vi "Example_GameWithVisual.vi"() -> ()   [LabVIEW 2015]
uses:
  TronviewGame/Game/GameResult.ctl
  TronviewGame/Board/BoardSize.ctl
  TronviewPresentation/BoardDisplay/BoardDisplay.lvclass
  TronviewGame/Game/Game.lvclass/Game.ctl
  TronviewGame/Game/GetGameRecorder.vi
  TronviewGame/GameRecorder/GameRecorder.lvclass
  TronviewGame/Board/Board.lvclass
  TronviewGame/Game/Game.lvclass
  TronviewGame/Player/Player.lvclass
  TronviewGame/TronviewGame.lvlib
panel:
  out "Board":u32[][](array[colorbox])=[[0, 0, 0, 0, 0, 0, 0, 0, 0, 0, 0, 0, 0, 0, 0, 0, 0, 0], [0, 16448250, 16448250, 16448250, 16448250, 16448250, 16448250, 16448250, 16448250, 16448250, 16448250, 16448250, 16448250, 16448250, 16448250, 16448250, 16448250, 0], [0, 16448250, 16448250, 16448250, 16448250, 16448250, 16448250, 16448250, 16448250, 16448250, 16448250, 16448250, 16448250, 16448250, 16448250, 16448250, 16448250, 0], [0, 16448250, 16448250, 16722502, 16448250, 16448250, 16448250, 16448250, 16448250, 16448250, 16448250, 16448250, 16448250, 16448250, 16448250, 16448250, 16448250, 0], [0, 16448250, 16448250, 16448250, 16448250, 16448250, 16448250, 16448250, 16448250, 16448250, 16448250, 16448250, 16448250, 16448250, 16448250, 16448250, 16448250, 0], [0, 16448250, 16448250, 16448250, 16448250, 16448250, 16448250, 16448250, 16448250, 16448250, 16448250, 16448250, 16448250, 16448250, 16448250, 16448250, 16448250, 0], [0, 16448250, 16448250, 16448250, 16448250, 16448250, 16448250, 16448250, 16448250, 16448250, 16448250, 16448250, 16448250, 16448250, 16448250, 16448250, 16448250, 0], [0, 16448250, 16448250, 16448250, 16448250, 16448250, 16448250, 16448250, 16448250, 16448250, 16448250, 16448250, 16448250, 16448250, 16448250, 16448250, 16448250, 0], [0, 16448250, 16448250, 16448250, 16448250, 16448250, 16448250, 16448250, 16448250, 16448250, 16448250, 16448250, 16448250, 16448250, 16448250, 16448250, 16448250, 0], [0, 16448250, 16448250, 16448250, 16448250, 16448250, 16448250, 16448250, 16448250, 16448250, 16448250, 16448250, 16448250, 16448250, 16448250, 16448250, 16448250, 0], [0, 16448250, 16448250, 16448250, 16448250, 16448250, 16448250, 16448250, 16448250, 16448250, 16448250, 16448250, 16448250, 16448250, 16448250, 16448250, 16448250, 0], [0, 16448250, 16448250, 16448250, 16448250, 16448250, 16448250, 16448250, 16448250, 16448250, 16448250, 16448250, 16448250, 16448250, 16448250, 16448250, 16448250, 0], [0, 16448250, 16448250, 16448250, 16448250, 16448250, 16448250, 16448250, 16448250, 16448250, 16448250, 16448250, 16448250, 16448250, 16448250, 16448250, 16448250, 0], [0, 16448250, 16448250, 16448250, 16448250, 16448250, 16448250, 16448250, 16448250, 16448250, 16448250, 16448250, 16448250, 16448250, 16448250, 16448250, 16448250, 0], [0, 16448250, 16448250, 16448250, 16448250, 16448250, 16448250, 16448250, 16448250, 16448250, 16448250, 16448250, 16448250, 16448250, 16448250, 16448250, 16448250, 0], [0, 16448250, 16448250, 16448250, 16448250, 16448250, 16448250, 16448250, 16448250, 16448250, 16448250, 16448250, 16448250, 16448250, 16448250, 2143232, 16448250, 0], [0, 16448250, 16448250, 16448250, 16448250, 16448250, 16448250, 16448250, 16448250, 16448250, 16448250, 16448250, 16448250, 16448250, 16448250, 16448250, 16448250, 0], [0, 0, 0, 0, 0, 0, 0, 0, 0, 0, 0, 0, 0, 0, 0, 0, 0, 0]]
  out "Array 2":picture[][](array[picture])
  out "error out":errorcluster
  in  "error in (no error)":errorcluster
  out "Finished?":bool
  out "GameResult":T1
  in  "IterationDelay (ms)":u32=10
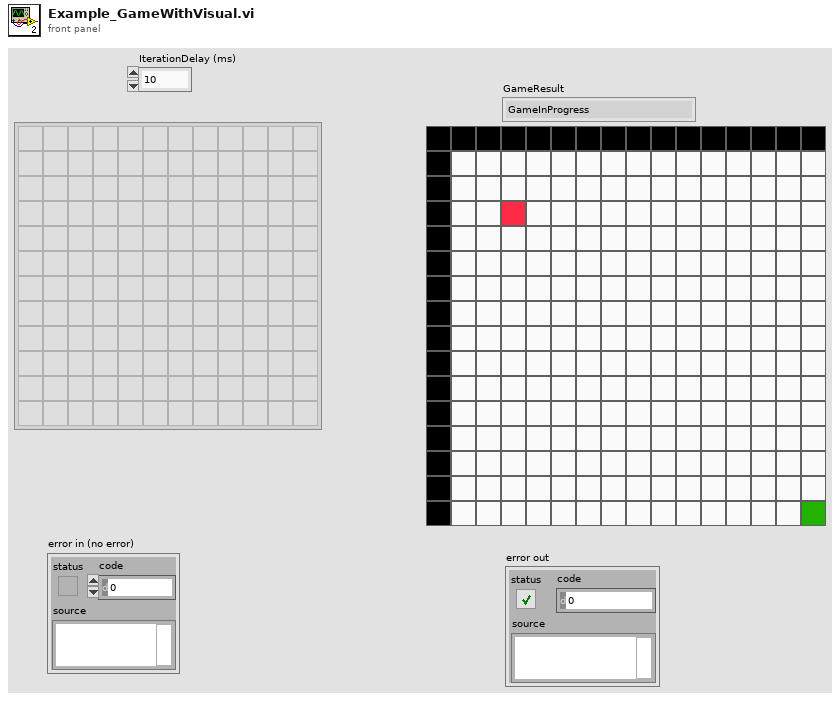
[diagram p1: front panel]
types:
  T1 = typedef "TronviewGame.lvlib/Game.lvclass/GameResult.ctl" = enum16{"GameInProgress", "Draw", "Player1Won", "Player2Won"}
  T2 = typedef "TronviewGame.lvlib/Board.lvclass/BoardSize.ctl" = cluster{"Columns":u16, "Rows":u16}
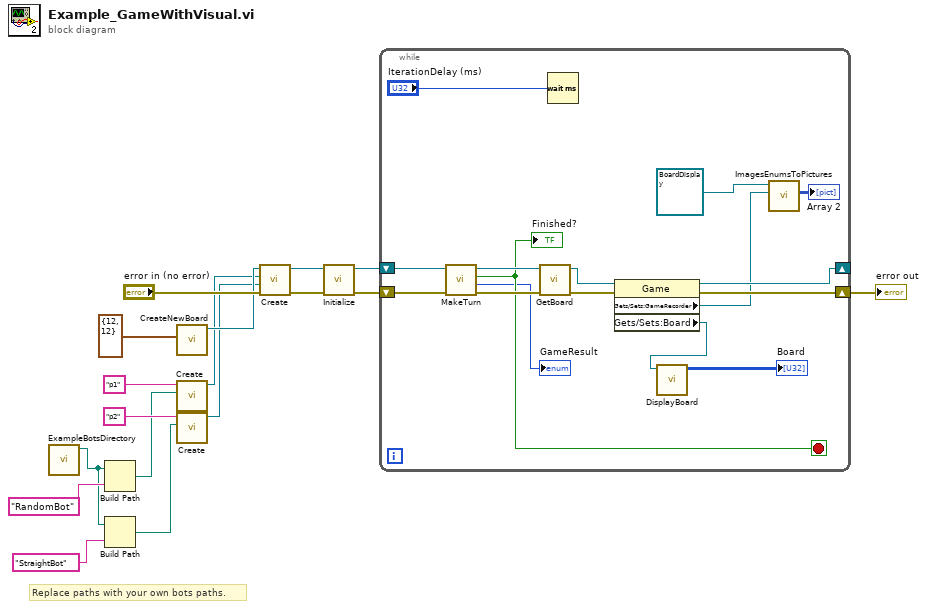
[diagram p0: block diagram]
diagram:
  # "Replace paths with your own bots paths."
  n1 = call "ExampleBotsDirectory.vi"() -> ("stripped path"=w7:path)  [unwired: 11 in]
  n2 = Build Path(base path=w7, name or relative path="RandomBot") -> (appended path=w4:path)
  n3 = Build Path(base path=w7, name or relative path="StraightBot") -> (appended path=w5:path)
  n4 = call "CreateNewBoard.vi"("Size"=T2 {"Columns"=12, "Rows"=12}) -> ("Board out"=w3:refnum<class "Board.lvclass">)  [unwired: 9 in, 1 out]
  n5 = call "Create.vi"("PlayerFolder"=w4, "PlayerName"="p1") -> ("Player out"=w2:refnum<class "Player.lvclass">)  [unwired: 8 in, 1 out]
  n6 = call "Create.vi"("PlayerFolder"=w5, "PlayerName"="p2") -> ("Player out"=w1:refnum<class "Player.lvclass">)  [unwired: 8 in, 1 out]
  n7 = call "Create.vi"("error in (no error)"="error in (no error)", "Player2"=w1, "Player1"=w2, "Board"=w3) -> ("error out"=w16:errorcluster, "Game out"=w17:refnum<class "Game.lvclass">)  [unwired: 6 in]
  n8 = call "Initialize.vi"("error in (no error)"=w16, "Game in"=w17) -> ("error out"=w14:errorcluster, "Game out"=w15:refnum<class "Game.lvclass">)  [unwired: 8 in]
  n9 = while {
    shift-right: [w24] -> _
    shift-left: w15 -> [w33]
    shift-right: [w23] -> w13
    shift-left: w14 -> [w32]
    stop <- w28 stop-if-true
    n10 = call "MakeTurn.vi"("error in (no error)"=w32, "Game in"=w33) -> ("error out"=w30:errorcluster, "GameResult"=→"GameResult":T1, "Finished?"=w28:bool, "Game out"=w31:refnum<class "Game.lvclass">)  [unwired: 6 in]
    "Finished?" <- w28
    n11 = call "GetBoard.vi"("error in (no error)"=w30, "Game in"=w31) -> ("error out"=w26:errorcluster, "Game out"=w25:refnum<class "Game.lvclass">)  [unwired: 7 in, 1 out]
    n12 = Wait (ms)(milliseconds to wait="IterationDelay (ms)") -> ()  [unwired: 1 out]
    n13 = property class="Game"(reference=w25, error in=w26) -> (reference out=w24:refnum<class "Game.lvclass">, error out=w23:errorcluster, "Gets/Sets:GameRecorder"=w22:refnum<class "GameRecorder.lvclass">, "Gets/Sets:Board"=w18:refnum<class "Board.lvclass">)
    n14 = call "DisplayBoard.vi"("Board"=w18) -> ("Array"=→"Board":u32[][])  [unwired: 10 in]
    n15 = call "ImagesEnumsToPictures.vi"("GameRecorder"=w22, "BoardDisplay in"=refnum<class "BoardDisplay.lvclass"> refnum) -> ("Array 2"=→"Array 2":picture[][])  [unwired: 7 in, 2 out]
  }
  "error out" <- w13
